vi "Sol_Tierra_Luna.vi"() -> ()   [LabVIEW 2016]
panel:
  out "Position:Top 2":i32
  out "Position:Left 2":i32
  out "Up":i32
  out "Left":i32
  in  "y":dbl=100.0
  out "Waveform Chart":cluster{i32, i32}(graph)
  out "Numeric Control":dbl
  out "Tierra":bool
  in  "Stop Button":bool
  out "Position:Top":i32
  out "Position:Left":i32
  in  "Posición Horizontal":i32(slide) scale=0.0..100.0
  in  "Posición Vertical":i32(slide) scale=0.0..100.0
  out "Sol":bool
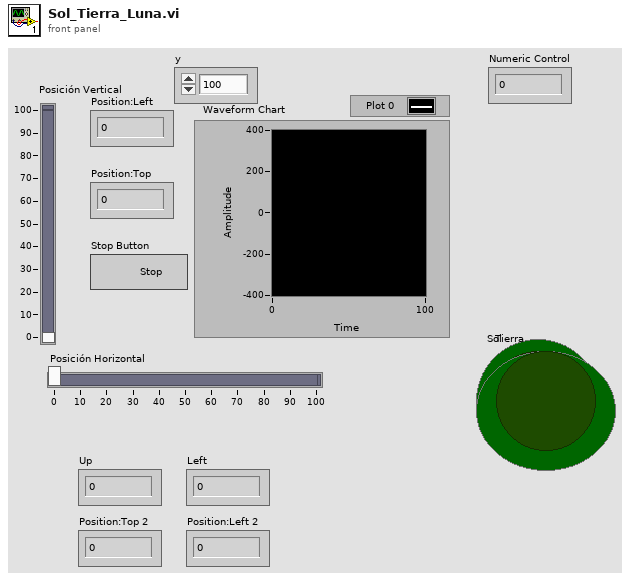
[diagram p1: front panel]
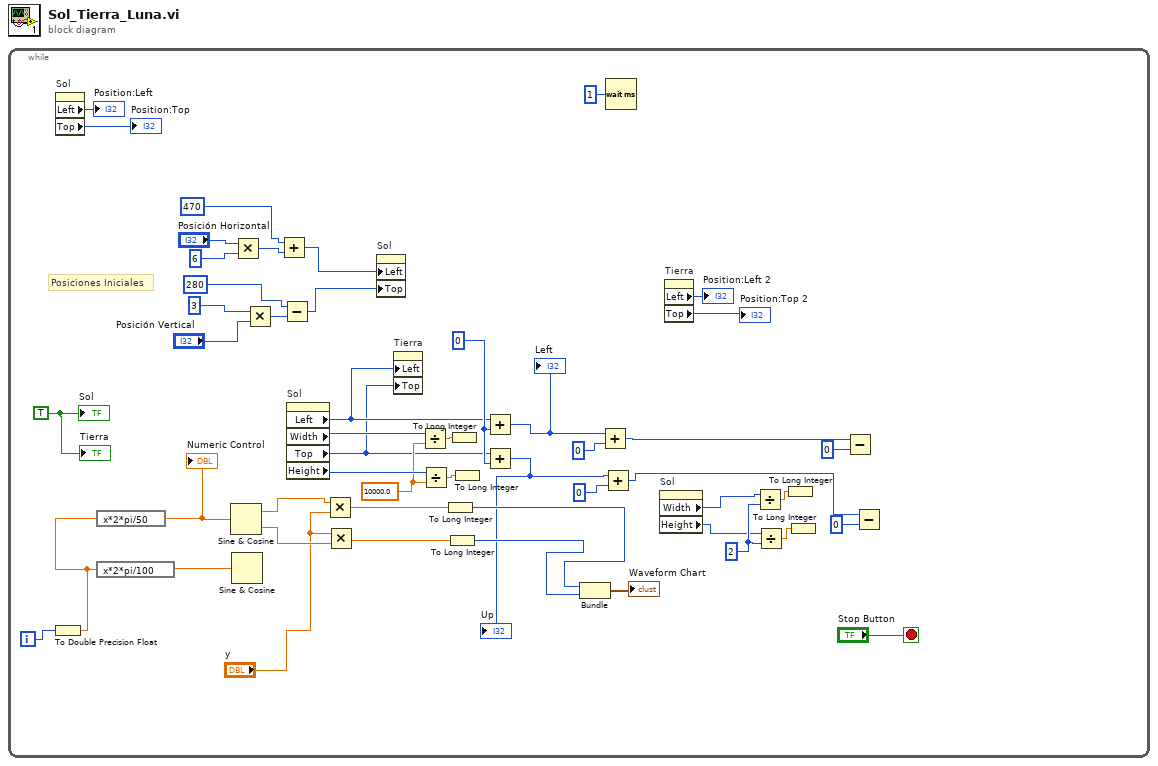
[diagram p0: block diagram]
diagram:
  n1 = while {
    i -> [w33]
    stop <- "Stop Button" stop-if-true
    w6 = 10000.0 ("y")
    w5 = 0 ("y")
    w18 = u32 2 ("y")
    w36 = TRUE ("Sol")
    # "Posiciones Iniciales"
    n2 = To Double Precision Float(number=w33) -> (double precision float=w32:dbl)
    n3 = property on="Sol" class="Bool (strict)"() -> ("Left"=→"Position:Left":i32, "Top"=→"Position:Top":i32)  [unwired: 2 in, 2 out]
    n4 = expression code="x*2*pi/50"(w32) -> (w34:dbl)
    "Numeric Control" <- w34
    n5 = expression code="x*2*pi/100"(w32) -> (w35:dbl)
    n6 = Sine & Cosine(0:w34) -> (1:w31:dbl, 2:w30:dbl)
    n7 = Sine & Cosine(0:w35) -> ()  [unwired: 2 out]
    n8 = Multiply(x="Posición Horizontal", y=6) -> (x*y=w37:i32)
    n9 = Multiply(x=3, y="Posición Vertical") -> (x*y=w46:i32)
    n10 = Add(x=470 ("Position:Left"), y=w37) -> (x+y=w39:i32)
    n11 = Subtract(x=280 ("Position:Top"), y=w46) -> (x-y=w40:i32)
    n12 = property on="Sol" class="Bool (strict)"() -> ("Left"=w4:i32, "Width"=w24:u32, "Top"=w3:i32, "Height"=w23:u32)  [unwired: 2 in, 2 out]
    n13 = Multiply(x=w31, y="y") -> (x*y=w29:dbl)
    n14 = Multiply(x="y", y=w30) -> (x*y=w28:dbl)
    n15 = property on="Sol" class="Bool (strict)"("Left"=w39, "Top"=w40) -> ()  [unwired: 2 in, 2 out]
    n16 = property on="Tierra" class="Bool (strict)"("Left"=w4, "Top"=w3) -> ()  [unwired: 2 in, 2 out]
    n17 = Divide(x=w24, y=w6) -> (x/y=w22:dbl)
    n18 = Divide(x=w23, y=w6) -> (x/y=w21:dbl)
    n19 = To Long Integer(number=w29) -> (32bit integer=w27:i32)
    n20 = To Long Integer(number=w28) -> (32bit integer=w26:i32)
    n21 = To Long Integer(number=w22) -> ()  [unwired: 1 out]
    n22 = To Long Integer(number=w21) -> ()  [unwired: 1 out]
    n23 = Add(x=w4, y=w5) -> (x+y=w19:i32)
    "Left" <- w19
    n24 = Add(x=w3, y=w5) -> (x+y=w20:i32)
    "Up" <- w20
    n25 = Bundle(w27, w26) -> (→"Waveform Chart":cluster{i32, i32})  [unwired: 1 in]
    n26 = Add(x=w19, y=0) -> (x+y=w15:i32)
    n27 = Add(x=w20, y=0) -> (x+y=w14:i32)
    n28 = Wait (ms)(milliseconds to wait=u32 1) -> ()  [unwired: 1 out]
    n29 = property on="Sol" class="Bool (strict)"() -> ("Width"=w10:u32, "Height"=w9:u32)  [unwired: 2 in, 2 out]
    n30 = property on="Tierra" class="Bool (strict)"() -> ("Left"=→"Position:Left 2":i32, "Top"=→"Position:Top 2":i32)  [unwired: 2 in, 2 out]
    n31 = Divide(x=w10, y=w18) -> (x/y=w17:dbl)
    n32 = Divide(x=w9, y=w18) -> (x/y=w16:dbl)
    n33 = To Long Integer(number=w17) -> ()  [unwired: 1 out]
    n34 = To Long Integer(number=w16) -> ()  [unwired: 1 out]
    n35 = Subtract(x=w15, y=0) -> ()  [unwired: 1 out]
    n36 = Subtract(x=w14, y=0) -> ()  [unwired: 1 out]
    "Sol" <- w36
    "Tierra" <- w36
  }
